vi "Sub Apply Frame Data.vi"(8 "error in (no error)":errorcluster, 11 "IDE simple in":refnum<class "Main Panel.lvclass">) -> (0 "error out":errorcluster, 3 "IDE simple out":refnum<class "Main Panel.lvclass">)   [LabVIEW 2018, in "Main Panel.lvlib" / "Main Panel.lvclass"]
uses:
  Main Panel.lvclass
  Main Panel.lvclass/Main Panel.ctl
  Frame Analizer/Data Parser.lvclass
  ScintillaNET/ScintillaNET.lvclass
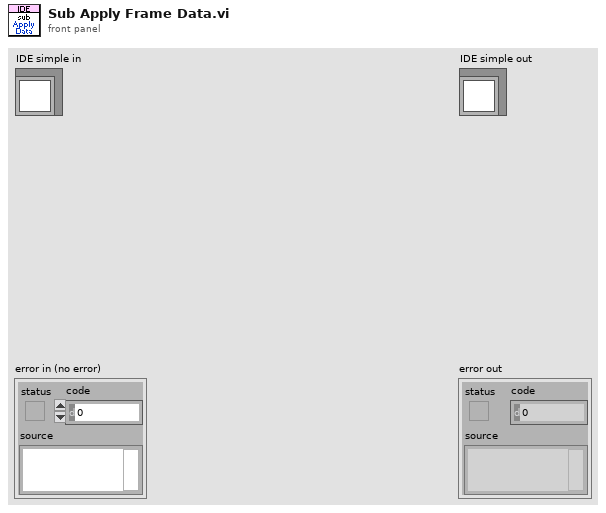
[diagram p1: front panel]
types:
  T1 = typedef "Data Parser.lvclass/frame data.ctl" = cluster{"Title":T2, "Basic Data":T3, "Sound":string, "<o> Data":T4, "<bp> Data":T5, "<c> Data":T6, "<w> Data":T7, "<i> Data Array":T8[], "<b> Data Array":T9[]}
  T2 = typedef "Data Parser.lvclass/frame title.ctl" = cluster{"Number":string, "Name":string}
  T3 = typedef "Data Parser.lvclass/frame basic data.ctl" = cluster{"Basic":cluster{"pic":string, "state":string, "wait":string, "next":string}, "Move":cluster{"dvx":string, "dvy":string, "dvz":string}, "Pic Center":cluster{"centerx":string, "centery":string}, "Skill":cluster{"hit_a":string, "hit_d":string, "hit_j":string, "hit_Fa":string, "hit_Ua":string, "hit_Da":string, "hit_Fj":string, "hit_Uj":string, "hit_Dj":string, "hit_ja":string}, "Mp":string}
  T4 = typedef "Data Parser.lvclass/frame o data.ctl" = cluster{"kind":string, "x":string, "y":string, "action":string, "dvx":string, "dvy":string, "dvz":string, "oid":string, "facing":string}
  T5 = typedef "Data Parser.lvclass/frame bp data.ctl" = cluster{"x":string, "y":string}
  T6 = typedef "Data Parser.lvclass/frame c data.ctl" = cluster{"kind":string, "x":string, "y":string, "injury":string, "cover":string, "vaction":string, "aaction":string, "taction":string, "hurtable":string, "decrease":string, "fronthurtact":string, "backhurtact":string, "dircontrol":string, "throwvx":string, "throwvy":string, "throwvz":string, "throwinjury":string}
  T7 = typedef "Data Parser.lvclass/frame w data.ctl" = cluster{"kind":string, "x":string, "y":string, "weaponact":string, "dvx":string, "dvy":string, "dvz":string, "attacking":string, "cover":string}
  T8 = typedef "Data Parser.lvclass/frame i data.ctl" = cluster{"kind":string, "x":string, "y":string, "w":string, "h":string, "dvx":string, "dvy":string, "dvz":string, "fall":string, "arest":string, "vrest":string, "bdefend":string, "injury":string, "zwidth":string, "effect":string, "catchingact":string, "caughtact":string}
  T9 = typedef "Data Parser.lvclass/frame b data.ctl" = cluster{"kind":string, "x":string, "y":string, "w":string, "h":string}
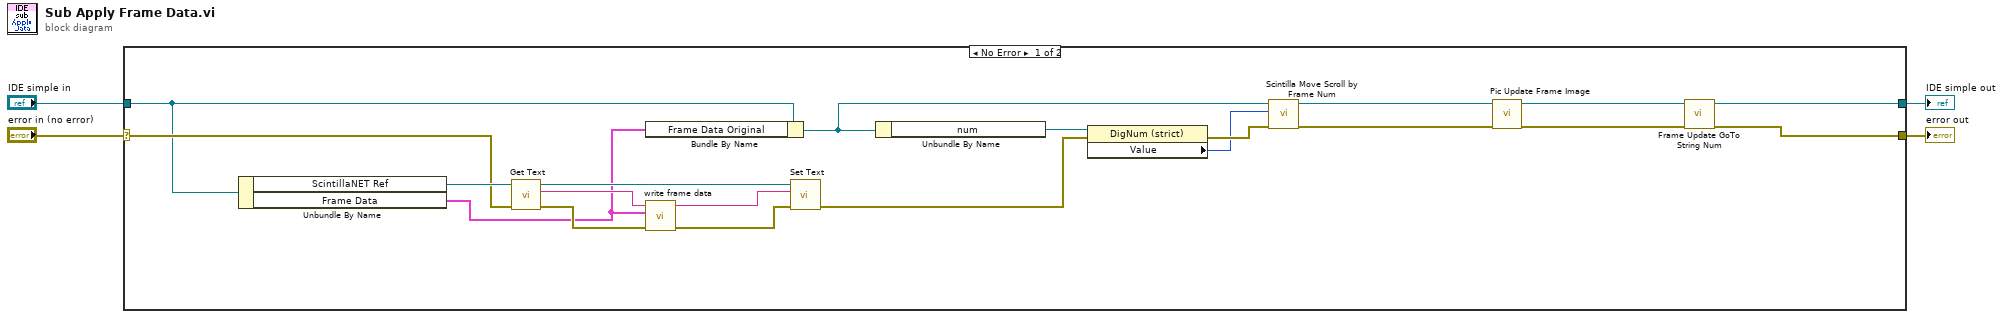
[diagram p0: block diagram]
diagram:
  n1 = case shown="No Error" "error in (no error)" {
    selector: "error in (no error)" -> [w18 w26]
    tunnel: [w11 w26] -> w3
    tunnel: [w12 w25] -> w1
    tunnel: "IDE simple in" -> [w16 w25]
    frame No Error {
      n2 = Unbundle By Name(w16) -> ("ScintillaNET Ref"=w24:refnum<class "ScintillaNET.lvclass">, "Frame Data"=w5:T1)
      n3 = call "Get Text.vi"("error in (no error)"=w18, "ScintillaNET in"=w24) -> ("error out"=w22:errorcluster, "Text"=w23:string, "ScintillaNET out"=w20:refnum<class "ScintillaNET.lvclass">)  [unwired: 7 in]
      n4 = Bundle By Name(cluster=w16, "Frame Data Original"=w5) -> (w6:refnum<class "Main Panel.lvclass">)
      n5 = call "write frame data.vi"("error in"=w22, "frame data"=w5, "file string in"=w23) -> ("error out"=w21:errorcluster, "file string out"=w19:string)  [unwired: 7 in]
      n6 = call "Set Text.vi"("error in (no error)"=w21, "Text"=w19, "ScintillaNET in"=w20) -> ("error out"=w15:errorcluster)  [unwired: 7 in, 1 out]
      n7 = Unbundle By Name(w6) -> ("num"=w17:refnum<vi>)
      n8 = property class="DigNum (strict)"(reference=w17, error in=w15) -> (error out=w14:errorcluster, "Value"=w13:u32)  [unwired: 1 out]
      n9 = call "Scintilla Move Scroll by Frame Num.vi"("error in (no error)"=w14, "Frame Number"=w13, "IDE simple in"=w6) -> ("error out"=w9:errorcluster, "IDE simple out"=w10:refnum<class "Main Panel.lvclass">)  [unwired: 7 in]
      n10 = call "Pic Update Frame Image.vi"("error in (no error)"=w9, "LF2R IDE in"=w10) -> ("error out"=w7:errorcluster, "LF2R IDE out"=w8:refnum<class "Main Panel.lvclass">)  [unwired: 8 in]
      n11 = call "Frame Update GoTo String Num.vi"("error in (no error)"=w7, "LF2R IDE in"=w8) -> ("error out"=w11:errorcluster, "LF2R IDE out"=w12:refnum<class "Main Panel.lvclass">)  [unwired: 8 in]
    }
    frame Error {
    }
  }
  "error out" <- w3
  "IDE simple out" <- w1
